vi "PXDAC4800_SessionStreamDeleteXD48.vi"(0 "SessionHandle":u32) -> (4 "Status":i32)   [LabVIEW 2016]
uses:
  PXDAC4800.dll
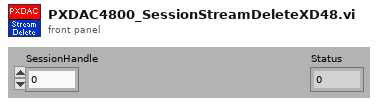
[diagram p1: front panel]
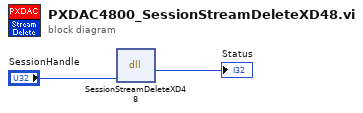
[diagram p0: block diagram]
diagram:
  n1 = dll-call lib="PXDAC4800.dll" fn="SessionStreamDeleteXD48"("Handle"="SessionHandle") -> (→"Status":i32)  [unwired: 4 in, 2 out]
